vi "connectSubDataPublish.vi"(8 "error in (no error)":errorcluster, 11 "MiddlewareSVThisComponent in":refnum<class "MiddlewareSVThisComponent.lvclass">) -> (0 "error out":errorcluster, 3 "MiddlewareSVThisComponent out":refnum<class "MiddlewareSVThisComponent.lvclass">)   [LabVIEW 2015, in "MiddlewareSVThisComponent.lvclass"]
uses:
  MiddlewareSVThisComponent.lvclass
  ComponentTemplateCore/ComponentModel/ComponentModel/Typedefs/CommunicationConfig.ctl
  ComponentTemplateCore/ComponentModel/ComponentModel/Typedefs/SVProcessConfig.ctl
  Typedefs/SubDataSV.ctl
  ComponentTemplateCore/ComponentModel/ComponentModel/Middleware/Middleware.lvclass/Middleware.ctl
  MiddlewareSVThisComponent.lvclass/MiddlewareSVThisComponent.ctl
  Model/Target/Target/Target.lvclass
  <vilib>/Utility/Data Type/NI_Data Type.lvlib
  ComponentTemplateCore/ComponentModel/ComponentModel/Middleware/Middleware.lvclass
  Typedefs/EXATypedefs.lvlib
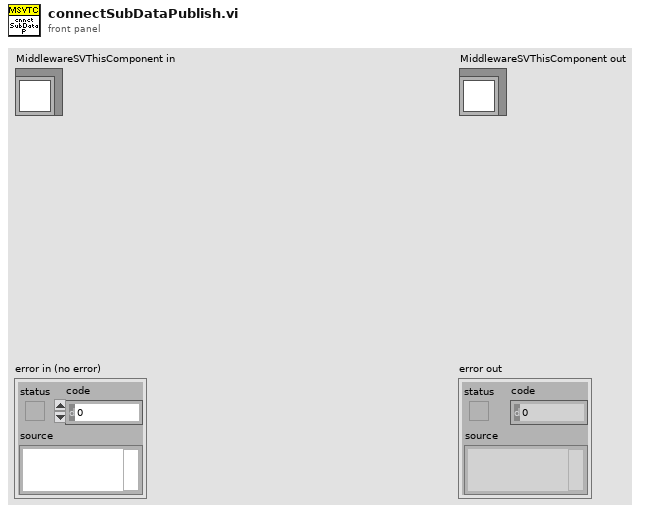
[diagram p1: front panel]
types:
  T1 = typedef "EXATypedefs.lvlib/SubDataSV.ctl" = enum16{"ClearError", "Disable", "Enable", "Exit", "GoToStandby", "HeartbeatIn", "Start"}
  T2 = typedef "SVProcessConfig.ctl" = cluster{"subDataProcessPrototype":string, "pubDataProcessPrototype":string, "commandProcessPrototype":string, "commandSVName":string}
  T3 = typedef "CommunicationConfig.ctl" = cluster{"hostComputerAddress":string, "ComponentAcronym":string, "InstanceIdentifier":i32}
  T4 = cluster{"Read Access":enum8{"Allowed", "Required", "None"}, "Write Access":enum8{"Allowed", "Required", "None"}}
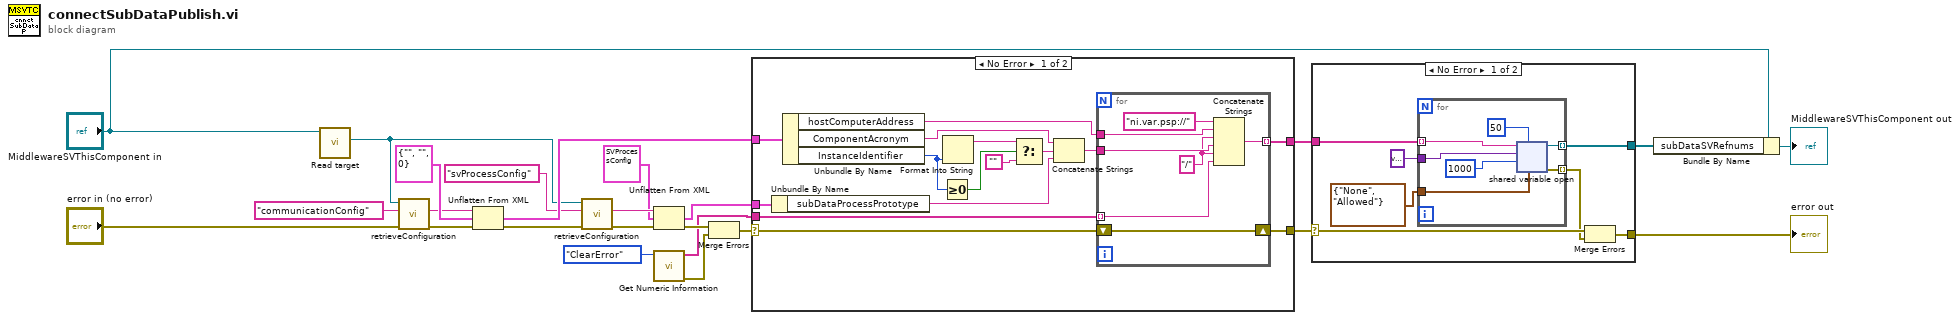
[diagram p0: block diagram]
diagram:
  n1 = call "Read target.vi"("Middleware in"="MiddlewareSVThisComponent in") -> ("target"=w2:refnum<class "Target.lvclass">)  [unwired: 9 in, 1 out]
  n2 = call-dynamic "retrieveConfiguration.vi"("error in (no error)"="error in (no error)", "dataName"="communicationConfig", "Target in"=w2) -> ("error out"=w18:errorcluster, "dataValueFromFile"=w19:string)  [unwired: 6 in, 1 out]
  n3 = Unflatten From XML(xml string=w19, type=T3 {"hostComputerAddress"="", "ComponentAcronym"="", "InstanceIdentifier"=0} ("sharedVariableLibrariesConfig"), error in (no error)=w18) -> (value=w14:T3, error out=w13:errorcluster)
  n4 = call-dynamic "retrieveConfiguration.vi"("error in (no error)"=w13, "dataName"="svProcessConfig", "Target in"=w2) -> ("error out"=w12:errorcluster, "dataValueFromFile"=w16:string)  [unwired: 6 in, 1 out]
  n5 = Unflatten From XML(xml string=w16, type=T2 {"subDataProcessPrototype"="SubDataSV", "pubDataProcessPrototype"="PubDataSV", "commandProcessPrototype"="CommandSV", "commandSVName"="Command"} ("svProcessConfig"), error in (no error)=w12) -> (value=w9:T2, error out=w11:errorcluster)
  n6 = call <vilib>:"Get Numeric Information.vi"("Variant"=SubDataSV."ClearError" ("SubDataSV")) -> ("error out"=w7:errorcluster, "Enum Names"=w8:string[])  [unwired: 7 in, 2 out]
  n7 = Merge Errors(w11, w7) -> (w17:errorcluster)
  n8 = case shown="No Error" w17 {
    selector: w17 -> [w34 w47]
    tunnel: [w39 _] -> w22
    tunnel: w14 -> [w37 _]
    tunnel: [w33 w47] -> w23
    tunnel: w8 -> [w27 _]
    tunnel: w9 -> [w26 _]
    frame No Error {
      n9 = Unbundle By Name(w26) -> ("subDataProcessPrototype"=w25:string)
      n10 = Unbundle By Name(w37) -> ("hostComputerAddress"=w36:string, "ComponentAcronym"=w38:string, "InstanceIdentifier"=w32:i32)
      n11 = Greater Or Equal To 0?(x=w32) -> (x >= 0?=w31:bool)
      n12 = Format Into String(w32) -> (resulting string=w30:string)  [unwired: 3 in, 1 out]
      n13 = Select(t=w30, s=w31, f="") -> (s? t:f=w28:string)
      n14 = Concatenate Strings(w38, w28, w25) -> (w35:string)
      n15 = for {
        tunnel: w36 -> [w45]
        tunnel: w35 -> [w44]
        tunnel: [w42] -> w39 mode=indexing
        shift-right: [w40] -> w33
        shift-left: w34 -> [w40]
        tunnel: w27 -> [w41] mode=indexing
        w43 = "/" ("string")
        n16 = Concatenate Strings("ni.var.psp://" ("string"), w45, w43, w44, w43, w41) -> (w42:string)
      }
    }
    frame Error {
    }
  }
  n17 = case shown="No Error" w23 {
    selector: w23 -> [w52 w62]
    tunnel: w22 -> [w53 _]
    tunnel: [w49 w62] -> w5
    tunnel: [w48 _] -> w21
    frame No Error {
      n18 = for {
        tunnel: T4 {"Read Access"=enum."None", "Write Access"=enum."Allowed"} ("access") -> [w61]
        tunnel: w53 -> [w60] mode=indexing
        tunnel: [w58] -> w48 mode=indexing
        tunnel: variant ("variant") -> [w57]
        tunnel: [w59] -> w51 mode=indexing
        n19 = shared-variable-open(w60, w57, w61, 1000 ("timeout ms"), u32 50 ("buffer size in elements")) -> (w58:refnum<k21>, w59:errorcluster)  [unwired: 1 in]
      }
      n20 = Merge Errors(w52, w51) -> (w49:errorcluster)
    }
    frame Error {
    }
  }
  "error out" <- w5
  n21 = Bundle By Name(cluster="MiddlewareSVThisComponent in", "subDataSVRefnums"=w21) -> (→"MiddlewareSVThisComponent out":refnum<class "MiddlewareSVThisComponent.lvclass">)
